vi "Hi_Port_DataSet.vi"(11 "InputStr":string) -> (3 "OutStr":string)   [LabVIEW 2018]
panel:
  in  "Output Current Max.Spec 18":string="*" caption="MAX"
  in  "Output Current Max.Spec 17":string="*" caption="MAX"
  in  "Output Current Max.Spec 16":string="*" caption="MAX"
  in  "Output Current Max.Spec 15":string="*" caption="MAX"
  in  "Output Current Max.Spec 14":string="*" caption="MAX"
  in  "Output Current Max.Spec 13":string="*" caption="MAX"
  in  "Output Current Max.Spec 12":string="*" caption="MAX"
  in  "Output Current Max.Spec 11":string="*" caption="MAX"
  in  "Output Current Max.Spec 10":string="*" caption="MAX"
  in  "Output Current Max.Spec 9":string="*" caption="MAX"
  in  "Output Current Max.Spec 8":string="*" caption="MAX"
  in  "Output Current Max.Spec 7":string="*" caption="MAX"
  in  "Output Current Max.Spec 6":string="*" caption="MAX"
  in  "Output Current Max.Spec 5":string="*" caption="MAX"
  in  "Output Current Max.Spec 4":string="*" caption="MAX"
  in  "Output Current Max.Spec 3":string="*" caption="MAX"
  in  "Output Current Max.Spec 2":string="*" caption="MAX"
  in  "Output Current Max.Spec":string="*" caption="MAX"
  in  "保存":bool
  in  "Exit":bool caption="停止"
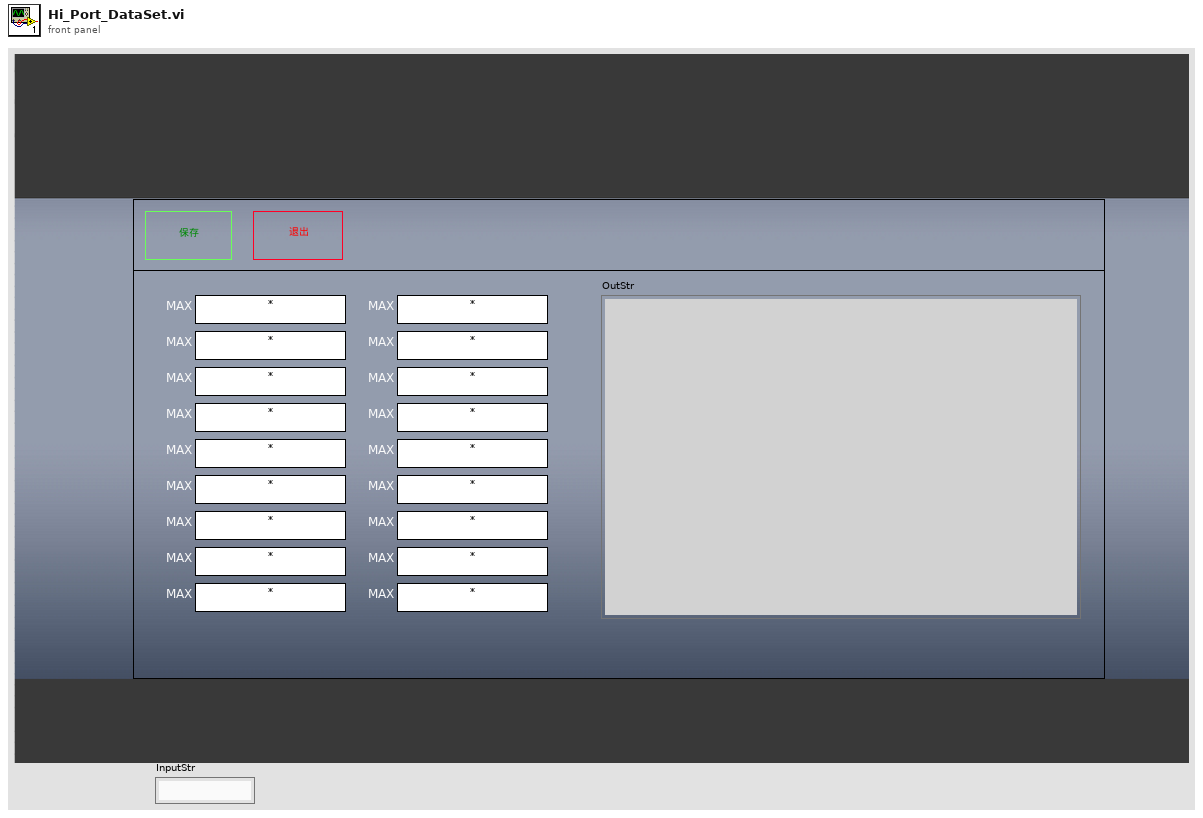
[diagram p1: front panel]
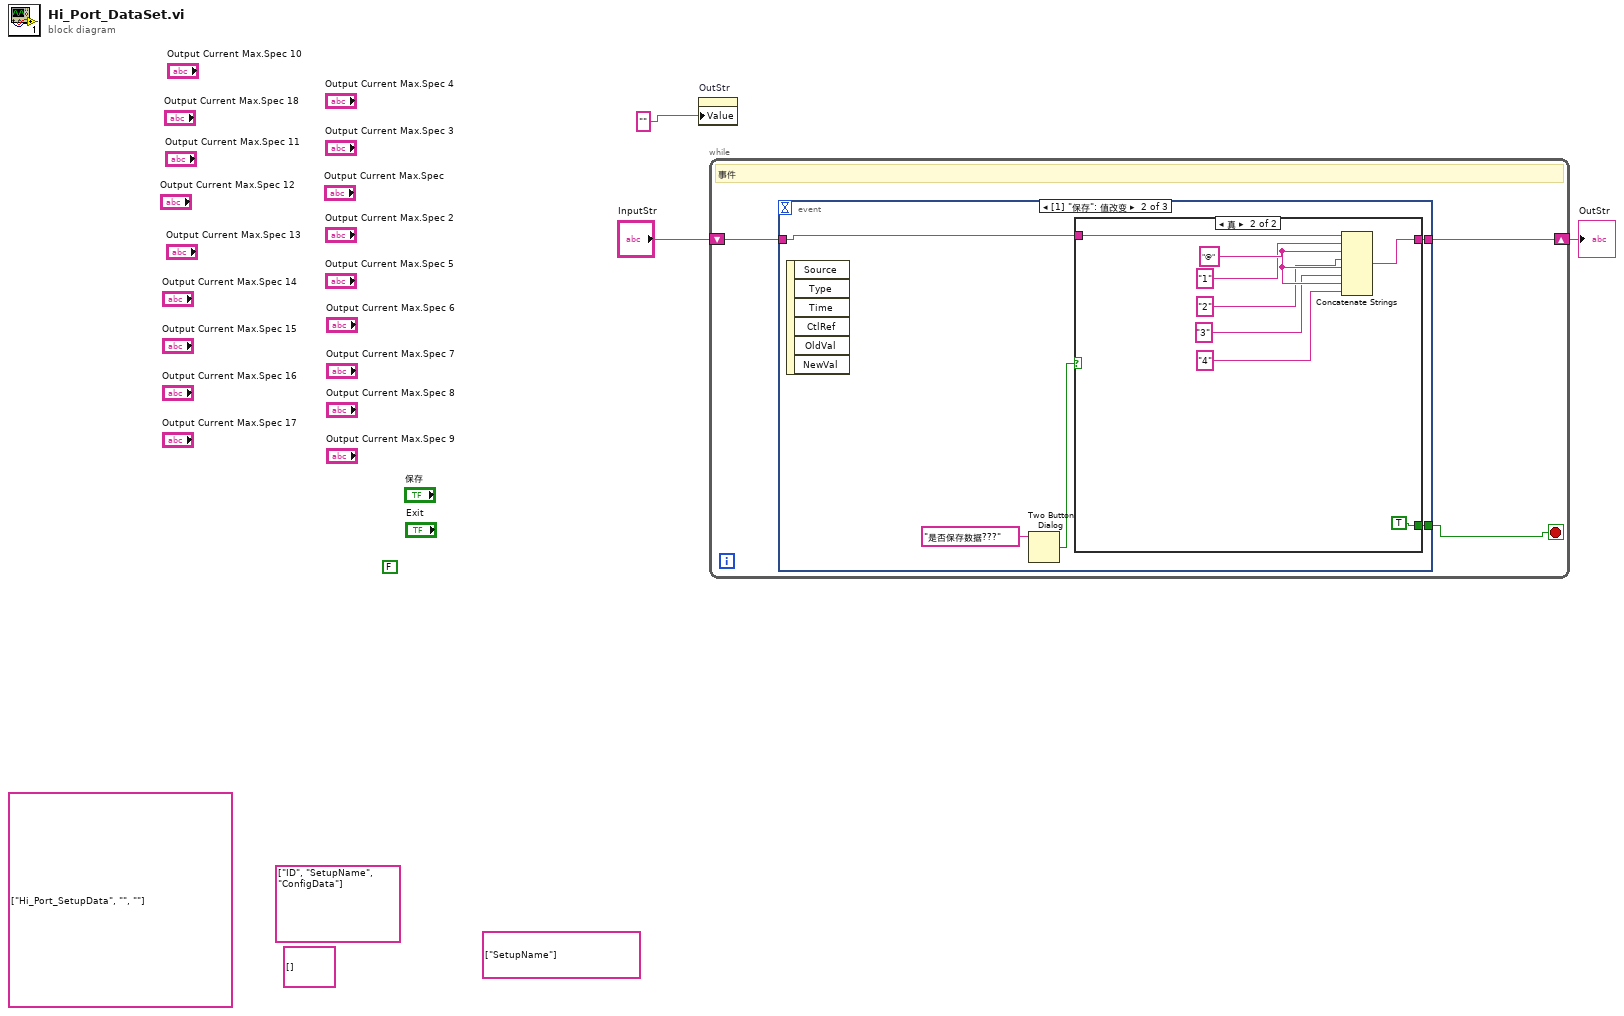
[diagram p0: block diagram]
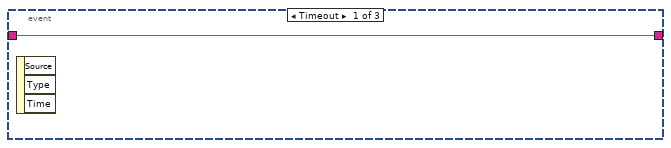
[diagram p2: hidden frame]
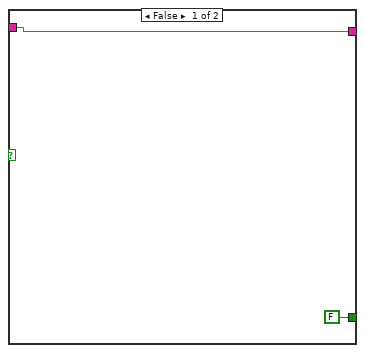
[diagram p3: hidden frame]
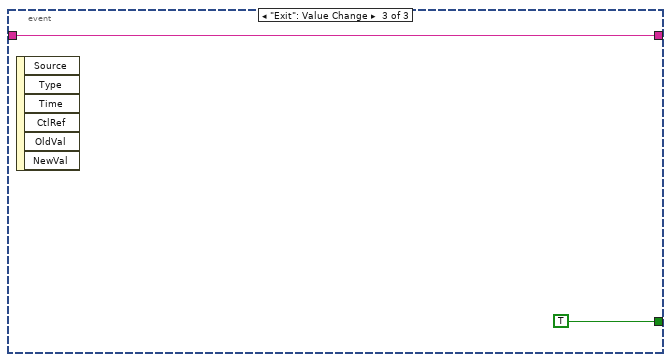
[diagram p4: hidden frame]
diagram:
  (unwired) string[] ["SetupName"]
  (unwired) string[][] [] ("项名")
  (unwired) string[] ["ID", "SetupName", "ConfigData"] ("Column Header Strings[]")
  (unwired) string[] ["Hi_Port_SetupData", "", ""]
  (unwired) FALSE ("exit")
  n1 = property on="OutStr" class="Str"("Value"="") -> ()  [unwired: 2 in, 2 out]
  n2 = while {
    shift-right: [w6] -> w3
    shift-left: "InputStr" -> [w5]
    stop <- w4 stop-if-true
    # "事件"
    n3 = event shown="[1] \"保存\": 值改变" {
      selector: _ -> [_ _ _]
      dyn-events: _ -> [_ _ _]
      timeout: _ -> [_ _ _]
      tunnel: [_ w10 TRUE] -> w4
      tunnel: [w7 w11 w23] -> w6
      tunnel: w5 -> [w7 w12 w23]
      event Timeout {
        n4 = event-data() -> ()  [unwired: 1 in, 3 out]
      }
      event "保存": Value Change {
        n5 = event-data() -> ()  [unwired: 1 in, 6 out]
        n6 = Two Button Dialog(message="是否保存数据???" ("消息")) -> (T button?=w8:bool)  [unwired: 2 in]
        n7 = case shown="真" w8 {
          tunnel: w12 -> [w14 w22]
          tunnel: [w14 w21] -> w11
          tunnel: [FALSE TRUE] -> w10
          frame False {
          }
          frame True {
            w20 = "@"
            n8 = Concatenate Strings(w22, "1" ("字符串"), w20, "2" ("字符串"), w20, "3" ("字符串"), w20, "4" ("字符串")) -> (w21:string)
          }
        }
      }
      event "Exit": Value Change {
        n9 = event-data() -> ()  [unwired: 1 in, 6 out]
      }
    }
  }
  "OutStr" <- w3
